vi "Node.Find.vi"(8 "error in (no error)":errorcluster, 10 "nodePath":string, 11 "System Def Root":refnum<k24>) -> (0 "error out":errorcluster, 1 "FindNode":bool, 2 "Node":refnum<k24>, 3 "System Def Root":refnum<k24>)   [LabVIEW 2015, in "Workspace.Obejct.Radio.lvlib"]
uses:
  Workspace.Obejct.Radio.lvlib
  NationalInstruments.VeriStand.SystemStorage
  NationalInstruments.VeriStand
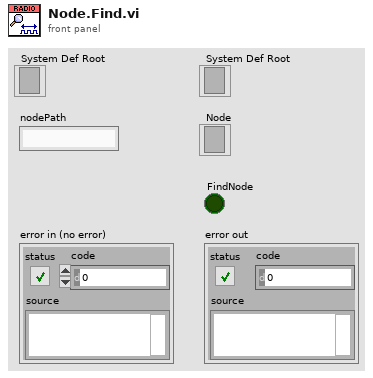
[diagram p1: front panel]
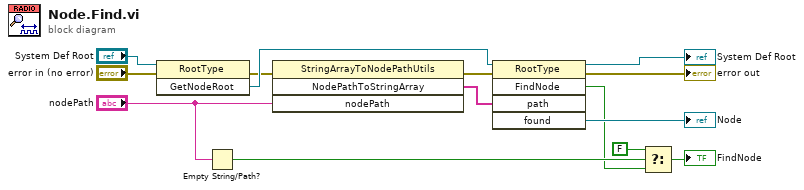
[diagram p0: block diagram]
diagram:
  n1 = invoke class="RootType" method="GetNodeRoot"(reference="System Def Root", error in="error in (no error)") -> (error out=w9:errorcluster, "GetNodeRoot"=w11:refnum<k24>)  [unwired: 1 in, 1 out]
  n2 = Empty String/Path?(string/path="nodePath") -> (empty?=w4:bool)
  n3 = invoke class="StringArrayToNodePathUtils" method="NodePathToStringArray"(error in=w9, "nodePath"="nodePath") -> (error out=w10:errorcluster, "NodePathToStringArray"=w8:string[])  [unwired: 2 in, 2 out]
  n4 = invoke class="RootType" method="FindNode"(reference=w11, error in=w10, "path"=w8) -> (reference out=→"System Def Root":refnum<k24>, error out=→"error out":errorcluster, "FindNode"=w3:bool, "found"=→"Node":refnum<k24>)  [unwired: 2 in, 1 out]
  n5 = Select(t=FALSE, s=w4, f=w3) -> (s? t:f=→"FindNode":bool)
